vi "niTuner Ready.vi"(8 "error in":errorcluster, 9 "timeout":dbl=1.0 format="%.2f", 11 "taskID in":i32 format="%.0x") -> (0 "error out":errorcluster, 2 "ready":bool, 3 "taskID out":i32 format="%.0x")   [LabVIEW 2011]
doc: "This VI returns the ready status of the PXI-5600 downconverter. The PXI-5600 is ready if the device is sufficiently settled on the requested frequency and all phase-locked loops (PLLs) are locked. Ready state is indicated by the <B>ready</B> output boolean and the STATUS light on the PXI-5600 downconverter front panel."
uses:
  nipxi5600u.dll
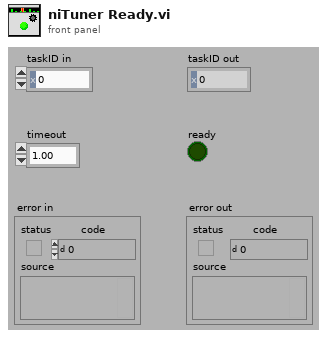
[diagram p1: front panel]
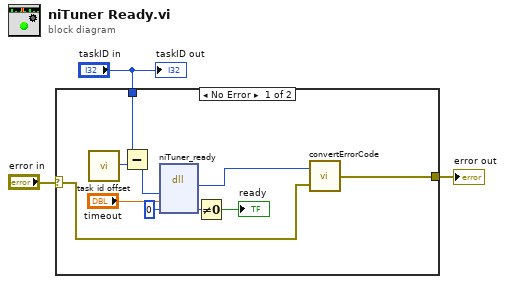
[diagram p0: block diagram]
diagram:
  n1 = case shown="No Error" "error in" {
    selector: "error in" -> [w6 w14]
    tunnel: [w5 w14] -> w2
    tunnel: "taskID in" -> [w4 _]
    frame No Error {
      n2 = call <instrlib>:"task id offset.vi"() -> ("taskID offset"=w12:i32)
      n3 = Subtract(x=w4, y=w12) -> (x-y=w13:i32)
      n4 = dll-call lib="nipxi5600u.dll" fn="niTuner_ready"("taskID"=w13, "timeout"="timeout", "ready"=u32 0) -> (w7:i32, "ready"=w9:u32)  [unwired: 5 in, 2 out]
      n5 = Not Equal To 0?(x=w9) -> (x != 0?=→"ready":bool)
      n6 = call <instrlib>:"convertErrorCode.vi"("error in"=w6, "error code"=w7) -> ("error out"=w5:errorcluster)
    }
    frame Error {
    }
  }
  "error out" <- w2
  "taskID out" <- "taskID in"
